vi "Copy Files.vi"(6 "Error Message in":string, 8 "Error In":errorcluster, 10 "Full App Name":string="PC Interface.exe", 11 "Server Files Cluster":T1) -> (0 "Error Out":errorcluster, 3 "Files Copied":bool, 4 "Error Message out":string)   [LabVIEW 2019]
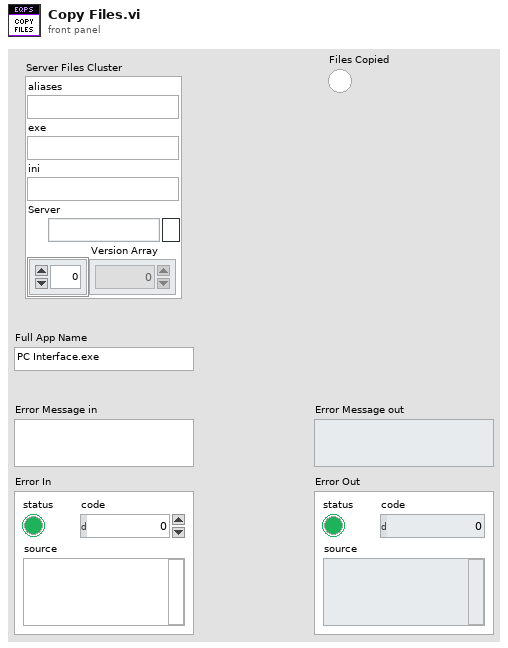
[diagram p1: front panel]
types:
  T1 = cluster{"aliases":string, "exe":string, "ini":string, "Server":path, "Version Array":i32[]}
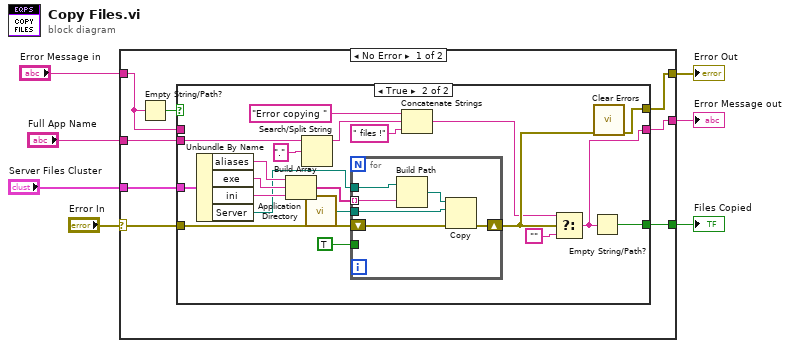
[diagram p0: block diagram]
diagram:
  n1 = case shown="No Error" "Error In" {
    selector: "Error In" -> [w11 w45]
    tunnel: [w12 w45] -> w6
    tunnel: [w14 w44] -> w5
    tunnel: "Error Message in" -> [w13 w44]
    tunnel: "Server Files Cluster" -> [w10 _]
    tunnel: [w9 _] -> w2
    tunnel: "Full App Name" -> [w8 _]
    frame No Error {
      n2 = Empty String/Path?(string/path=w13) -> (empty?=w15:bool)
      n3 = case shown="True" w15 {
        tunnel: [w17 w27] -> w14
        tunnel: w13 -> [w17 _]
        tunnel: [w16 w29] -> w12
        tunnel: w11 -> [w16 w26]
        tunnel: w10 -> [_ w36]
        tunnel: [_ w28] -> w9
        tunnel: w8 -> [_ w22]
        frame False {
        }
        frame True {
          n4 = Unbundle By Name(w36) -> ("aliases"=w33:string, "exe"=w35:string, "ini"=w34:string, "Server"=w24:path)
          n5 = Build Array(w33, w35, w34) -> (w32:string[])
          n6 = Search/Split String(string=w22, search string/char (-)=".") -> (substring before match=w20:string)  [unwired: 1 in, 2 out]
          n7 = call <vilib>:"Application Directory.vi"() -> ("Application Directory"=w37:path)
          n8 = for {
            tunnel: w37 -> [w38]
            tunnel: w32 -> [w42] mode=indexing
            shift-right: [w41] -> w25
            shift-left: w26 -> [w40]
            tunnel: TRUE ("overwrite (F)") -> [_]
            tunnel: w24 -> [w43]
            n9 = Build Path(base path=w43, name or relative path=w42) -> (appended path=w39:path)
            n10 = Copy(8:w40, 10:w38, 11:w39) -> (0:w41:errorcluster)  [unwired: 2 in, 2 out]
          }
          n11 = Concatenate Strings("Error copying ", w20, " files !") -> (w18:string)
          n12 = Select(t=w18, s=w25, f="") -> (s? t:f=w27:string)
          n13 = Empty String/Path?(string/path=w27) -> (empty?=w28:bool)
          n14 = call <vilib>:"Clear Errors.vi"("error in (no error)"=w25) -> ("error out"=w29:errorcluster)  [unwired: 5 in, 1 out]
        }
      }
    }
    frame Error {
    }
  }
  "Error Out" <- w6
  "Error Message out" <- w5
  "Files Copied" <- w2
